vi "bumper e.vi"() -> ()   [LabVIEW 2013]
uses:
  <vilib>/NXT/Block Support/NXT_InputPort.ctl
  <vilib>/NXT/Block Support/NXT_MessageMailbox.ctl
  <vilib>/NXT/Subs/MotorOutput.ctl
  <vilib>/NXT/Block Support/NXT_OutputPort.ctl
  <vilib>/NXT/Dual Mode Library/Display/drawNumber.vi
  <vilib>/NXT/Dual Mode Library/BT/BlueTooth_Write_Num.vi
  <vilib>/NXT/Dual Mode Library/Display/drawNumber_float.vi
  <vilib>/NXT/NXTIO Xnodes/NXTIONodeSubVIs/NXTStopMotors.vi
  <vilib>/NXT/NXTIO Xnodes/AddressXNode/NXTIOAddress.xnode
  <vilib>/NXT/NXTIO Xnodes/NXTIOXNode/NXTIO.xnode
  <vilib>/NXT/Subs/LVHSConnector.ctl
  <vilib>/NXT/LegoClasses/BrickReference/BrickReference.lvclass
panel:
  out "Case Accord. BJr.":i32
  out "touch right":bool
  out "touch left":bool
  in  "threshold steer":dbl=0.2
  out "norm dist":dbl
  out "right dist":i16
  out "left dist":i16
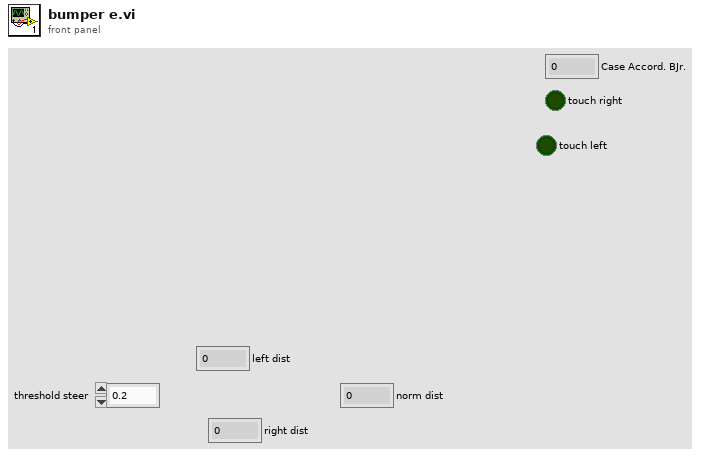
[diagram p1: front panel]
types:
  T1 = typedef "NXT_OutputPort.ctl" = u8
  T2 = typedef "NXT_MessageMailbox.ctl" = u8
  T3 = typedef "NXT_InputPort.ctl" = u32
  T4 = typedef "LVHSConnector.ctl" = refnum<class "BrickReference.lvclass">
  T5 = typedef "MotorOutput.ctl" = u8
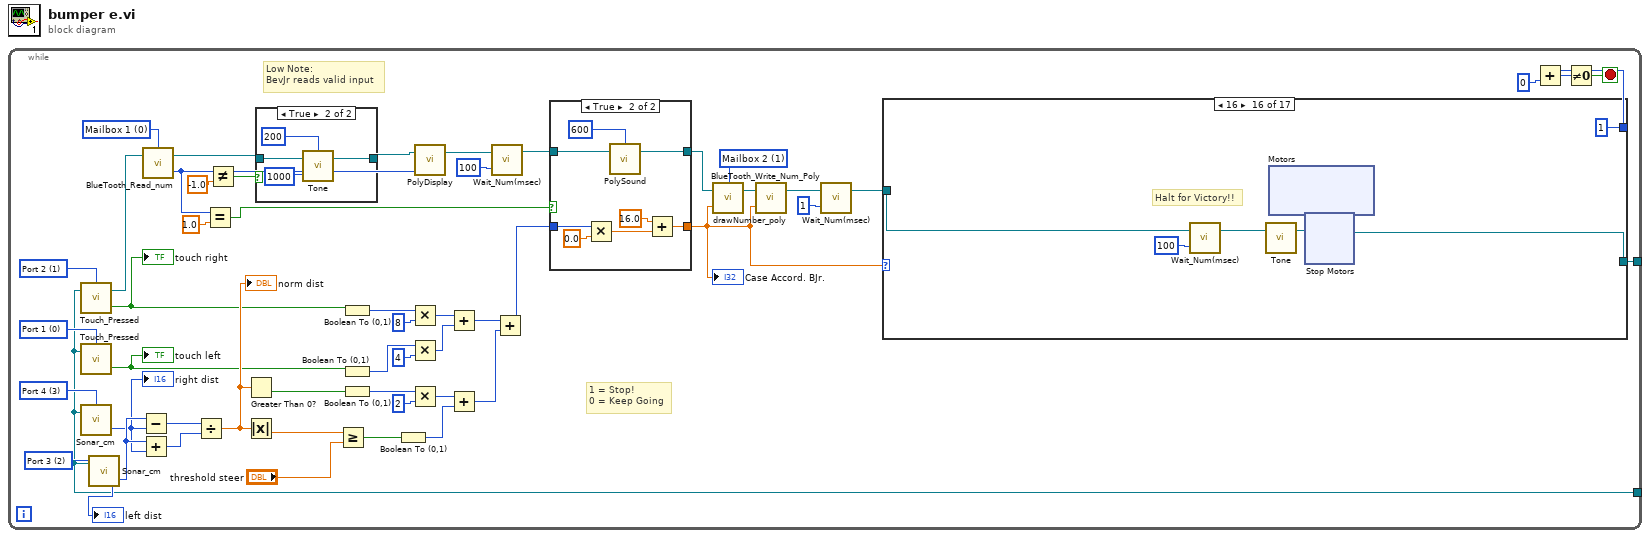
[diagram p0: block diagram]
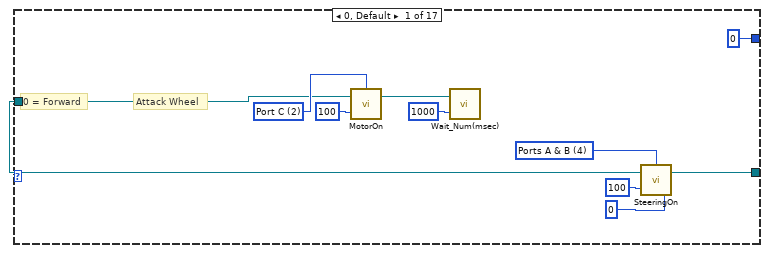
[diagram p3: hidden frame]
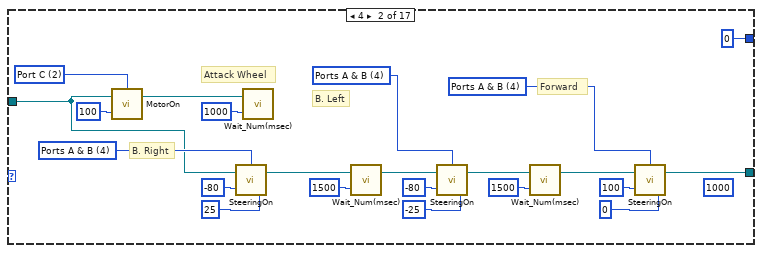
[diagram p4: hidden frame]
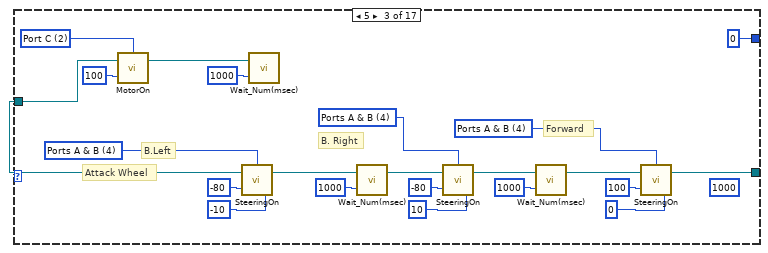
[diagram p5: hidden frame]
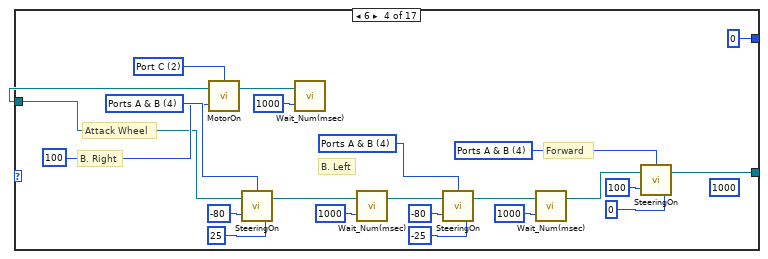
[diagram p6: hidden frame]
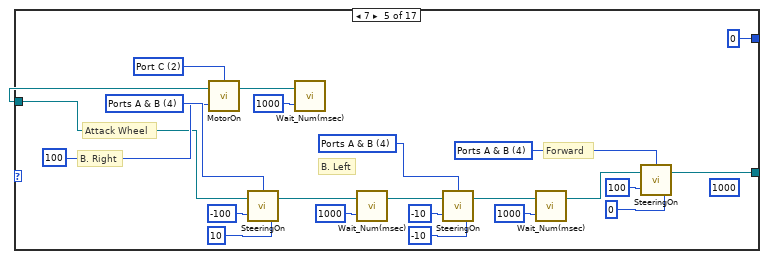
[diagram p7: hidden frame]
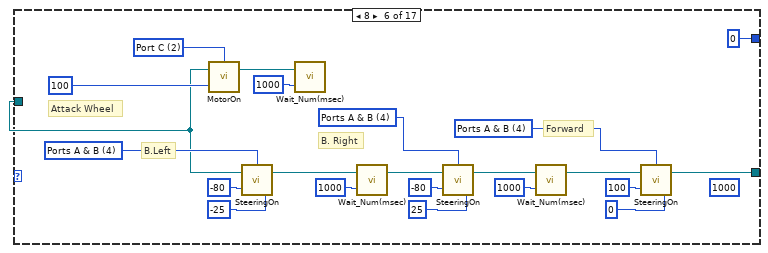
[diagram p8: hidden frame]
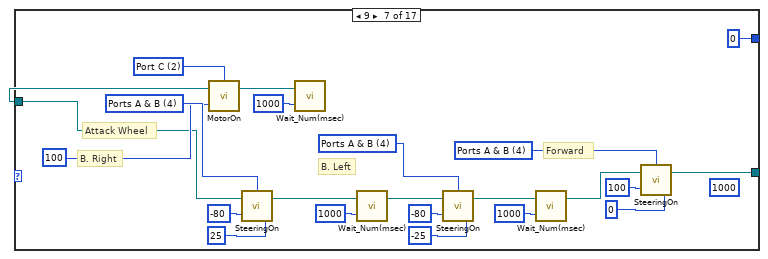
[diagram p9: hidden frame]
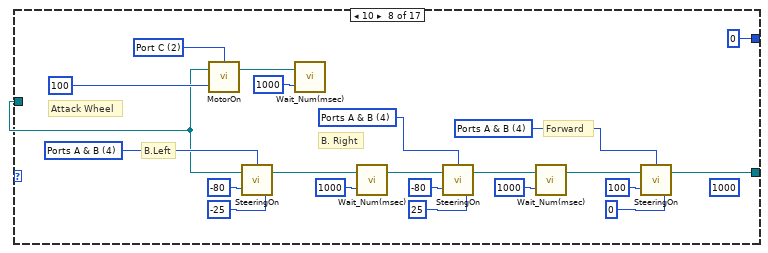
[diagram p10: hidden frame]
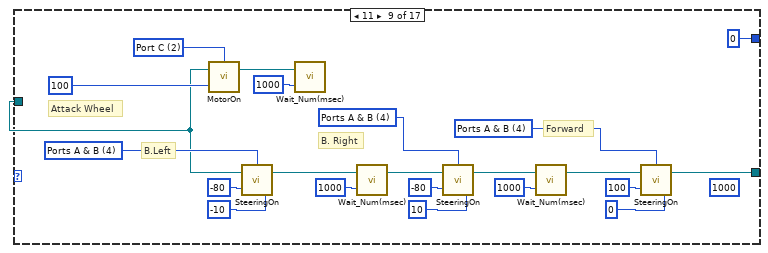
[diagram p11: hidden frame]
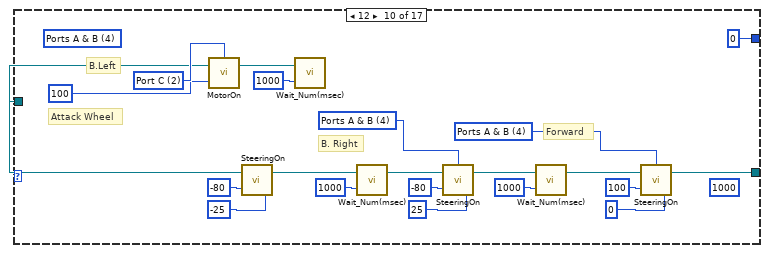
[diagram p12: hidden frame]
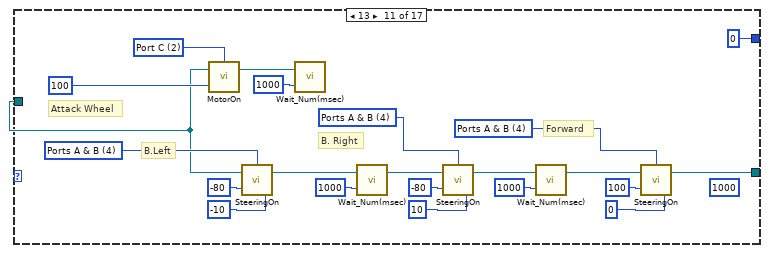
[diagram p13: hidden frame]
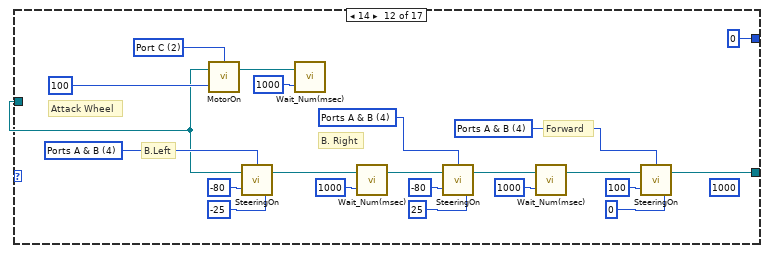
[diagram p14: hidden frame]
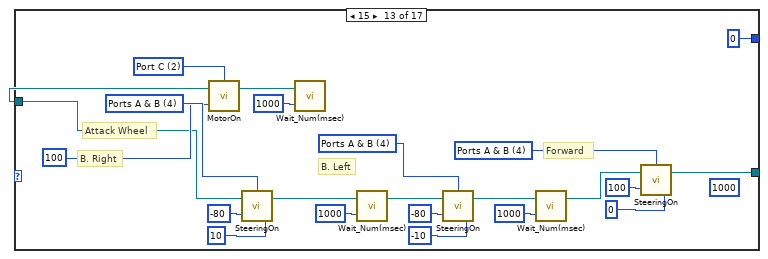
[diagram p15: hidden frame]
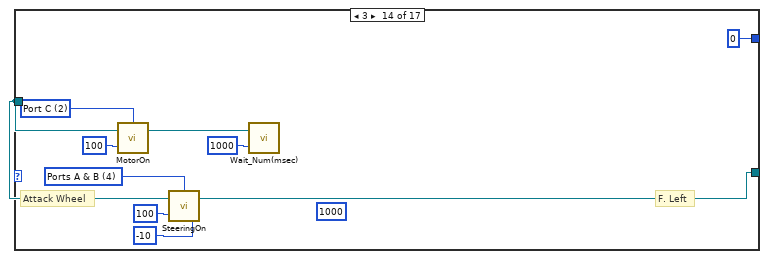
[diagram p16: hidden frame]
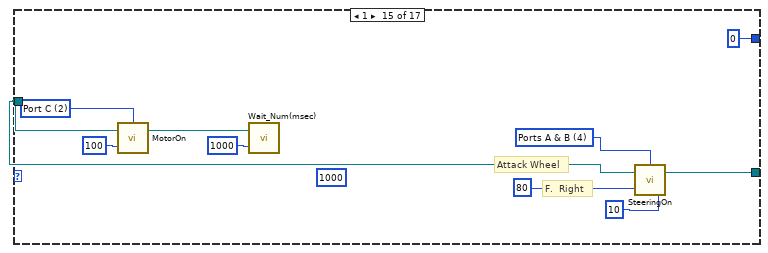
[diagram p17: hidden frame]
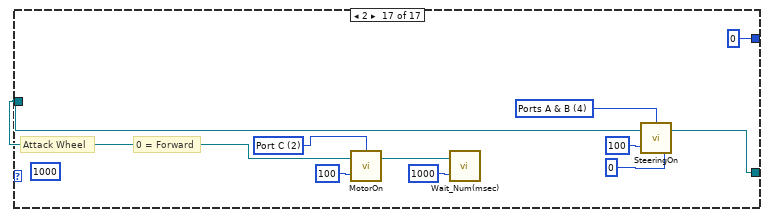
[diagram p18: hidden frame]
diagram:
  n1 = while {
    tunnel: [w20] -> _
    tunnel: [w14] -> _
    stop <- w22 stop-if-true
    w11 = T2 0 items=["Mailbox 1", "Mailbox 2", "Mailbox 3", "Mailbox 4", "Mailbox 5", "Mailbox 6", "Mailbox 7", "Mailbox 8", "Mailbox 9", "Mailbox 10"] ("Mailbox")
    w18 = T2 1 items=["Mailbox 1", "Mailbox 2", "Mailbox 3", "Mailbox 4", "Mailbox 5", "Mailbox 6", "Mailbox 7", "Mailbox 8", "Mailbox 9", "Mailbox 10"] ("Mailbox")
    w43 = T3 1 items=["Port 1", "Port 2", "Port 3", "Port 4"] ("Port (Port 1)")
    w44 = T3 0 items=["Port 1", "Port 2", "Port 3", "Port 4"] ("Port (Port 1)")
    w52 = T3 3 items=["Port 1", "Port 2", "Port 3", "Port 4"] ("Port (Port 4)")
    w53 = T3 2 items=["Port 1", "Port 2", "Port 3", "Port 4"] ("Port (Port 4)")
    # "Low Note:\nBevJr reads valid input"
    # "1 = Stop!\n0 = Keep Going"
    n2 = call <vilib>:"Sonar_cm.vi"("Port (Port 4)"=w53) -> ("Distance (cm)"=w51:i16, "NXT/EV3"=w20:T4)  [unwired: 2 in]
    "left dist" <- w51
    n3 = call <vilib>:"Touch_Pressed.vi"("NXT/EV3"=w20, "Port (Port 1)"=w43) -> ("Yes / No"=w29:bool, "NXT/EV3"=w10:T4)  [unwired: 1 in]
    "touch right" <- w29
    n4 = call <vilib>:"Touch_Pressed.vi"("NXT/EV3"=w20, "Port (Port 1)"=w44) -> ("Yes / No"=w30:bool)  [unwired: 1 in, 1 out]
    "touch left" <- w30
    n5 = call <vilib>:"Sonar_cm.vi"("NXT/EV3"=w20, "Port (Port 4)"=w52) -> ("Distance (cm)"=w50:i16)  [unwired: 1 in, 1 out]
    "right dist" <- w50
    n6 = Subtract(x=w51, y=w50) -> (x-y=w49:i16)
    n7 = Add(x=w51, y=w50) -> (x+y=w48:i16)
    n8 = call <vilib>:"BlueTooth_Read_num.vi"("NXT/EV3"=w10, "Mailbox"=w11) -> ("Message"=w4:i32, "NXT/EV3"=w3:T4)  [unwired: 1 in]
    n9 = Divide(x=w49, y=w48) -> (x/y=w45:dbl)
    "norm dist" <- w45
    n10 = Equal?(x=w4, y=1.0) -> (x = y?=w25:bool)
    n11 = Not Equal?(x=w4, y=-1.0) -> (x != y?=w5:bool)
    n12 = Greater Than 0?(x=w45) -> (x > 0?=w28:bool)
    n13 = Absolute Value(x=w45) -> (abs(x)=w47:dbl)
    n14 = case shown="True" w5 {
      tunnel: w3 -> [w54 w56]
      tunnel: [w54 w55] -> w2
      frame False {
      }
      frame True {
        n15 = call <vilib>:"Tone.vi"("Duration (500 ms)"=u16 1000, "NXT/EV3"=w56, "Tone (440 Hz)"=u16 200) -> ("NXT/EV3"=w55:T4)  [unwired: 1 in]
      }
    }
    n16 = Greater Or Equal?(x=w47, y="threshold steer") -> (x >= y?=w27:bool)
    n17 = Boolean To (0,1)(Boolean=w29) -> (0, 1=w38:i16)
    n18 = Boolean To (0,1)(Boolean=w30) -> (0, 1=w37:i16)
    n19 = Boolean To (0,1)(Boolean=w28) -> (0, 1=w42:i16)
    n20 = Boolean To (0,1)(Boolean=w27) -> (0, 1=w32:i16)
    n21 = Multiply(x=w38, y=i16 8) -> (x*y=w35:i16)
    n22 = Multiply(x=w37, y=i16 4) -> (x*y=w34:i16)
    n23 = Multiply(x=w42, y=i16 2) -> (x*y=w33:i16)
    n24 = call-poly <vilib>:"PolyDisplay.vi"("number"=w4, "NXT/EV3"=w2) -> ("NXT/EV3"=w12:T4)  [unwired: 2 in]
    n25 = Add(x=w35, y=w34) -> (x+y=w36:i16)
    n26 = Add(x=w33, y=w32) -> (x+y=w31:i16)
    n27 = call <vilib>:"Wait_Num(msec).vi"("Time (100 msec)"=u32 100, "NXT/EV3"=w12) -> ("NXT/EV3"=w9:T4)  [unwired: 2 in]
    n28 = Add(x=w36, y=w31) -> (x+y=w21:i16)
    n29 = case shown="True" w25 {
      tunnel: w21 -> [w376 w382]
      tunnel: [w376 w377] -> w7
      tunnel: w9 -> [w375 w381]
      tunnel: [w375 w380] -> w16
      frame False {
      }
      frame True {
        n30 = Multiply(x=w382, y=0.0) -> (x*y=w379:dbl)
        n31 = call-poly <vilib>:"PolySound.vi"("NXT/EV3"=w381, "Tone (440 Hz)"=u16 600) -> ("NXT/EV3"=w380:T4)  [unwired: 2 in]
        n32 = Add(x=16.0, y=w379) -> (x+y=w377:dbl)
      }
    }
    "Case Accord. BJr." <- w7
    n33 = call-poly <vilib>:"BlueTooth_Write_Num_Poly.vi"("Message"=w7, "NXT/EV3"=w16, "Mailbox"=w18) -> ("NXT/EV3"=w19:T4)  [unwired: 1 in]
    n34 = call-poly <vilib>:"drawNumber_poly.vi"("number"=w7, "NXT/EV3"=w19) -> ("NXT/EV3"=w1:T4)  [unwired: 2 in]
    n35 = call <vilib>:"Wait_Num(msec).vi"("Time (100 msec)"=u32 1, "NXT/EV3"=w1) -> ("NXT/EV3"=w15:T4)  [unwired: 2 in]
    n36 = case shown="16" w7 {
      tunnel: [w66 w84 w97 w119 w141 w172 w185 w207 w229 w251 w272 w294 w317 w339 w349 w356 w372] -> w14
      tunnel: w15 -> [w59 w69 w91 w113 w135 w157 w179 w201 w223 w245 w267 w288 w310 w332 w342 w352 w366]
      tunnel: [0 ("Steering (100)") 0 ("Steering (100)") 0 ("Steering (100)") 0 ("Steering (100)") 0 ("Steering (100)") 0 ("Steering (100)") 0 ("Steering (100)") 0 ("Steering (100)") 0 ("Steering (100)") 0 ("Steering (100)") 0 ("Steering (100)") 0 ("Steering (100)") 0 ("Steering (100)") 0 ("Steering (100)") 0 ("Steering (100)") 1 ("Steering (100)") 0 ("Steering (100)")] -> w13
      frame 0, Default {
        w64 = T5 2 items=["Port A"=0, "Port B"=1, "Port C"=2, "Ports A & B"=4, "Ports A & C"=5, "Ports B & C"=6, "All Ports"=3] ("Output Ports (A & B)")
        w65 = T5 4 items=["Port A"=0, "Port B"=1, "Port C"=2, "Ports A & B"=4, "Ports A & C"=5, "Ports B & C"=6, "All Ports"=3] ("Output Ports (A & B) 5")
        # "Attack Wheel"
        # "0 = Forward"
        n37 = call <vilib>:"MotorOn.vi"("Power (75)"=100, "NXT/EV3"=w59, "Output Port (All Ports)"=w64) -> ("NXT/EV3"=w62:T4)  [unwired: 1 in]
        n38 = call <vilib>:"Wait_Num(msec).vi"("Time (100 msec)"=u32 1000, "NXT/EV3"=w62) -> ()  [unwired: 2 in, 1 out]
        n39 = call <vilib>:"SteeringOn.vi"("Power (75)"=100, "Steering (100)"=0, "NXT/EV3"=w59, "Output Ports (A & B)"=w65) -> ("NXT/EV3"=w66:T4)
      }
      frame 4 {
        (unwired) u16 1000 ("Duration (500 ms)")
        w74 = T5 2 items=["Port A"=0, "Port B"=1, "Port C"=2, "Ports A & B"=4, "Ports A & C"=5, "Ports B & C"=6, "All Ports"=3] ("Output Ports (A & B)")
        w81 = T5 4 items=["Port A"=0, "Port B"=1, "Port C"=2, "Ports A & B"=4, "Ports A & C"=5, "Ports B & C"=6, "All Ports"=3] ("Output Ports (A & B) 15")
        w82 = T5 4 items=["Port A"=0, "Port B"=1, "Port C"=2, "Ports A & B"=4, "Ports A & C"=5, "Ports B & C"=6, "All Ports"=3] ("Output Port (All Ports) 6")
        w83 = T5 4 items=["Port A"=0, "Port B"=1, "Port C"=2, "Ports A & B"=4, "Ports A & C"=5, "Ports B & C"=6, "All Ports"=3] ("Output Ports (A & B) 16")
        # "Attack Wheel"
        # "Forward"
        # "B. Left"
        # "B. Right"
        n40 = call <vilib>:"MotorOn.vi"("Power (75)"=100, "NXT/EV3"=w69, "Output Port (All Ports)"=w74) -> ("NXT/EV3"=w72:T4)  [unwired: 1 in]
        n41 = call <vilib>:"SteeringOn.vi"("Power (75)"=-80, "Steering (100)"=25, "NXT/EV3"=w69, "Output Ports (A & B)"=w83) -> ("NXT/EV3"=w80:T4)
        n42 = call <vilib>:"Wait_Num(msec).vi"("Time (100 msec)"=u32 1000, "NXT/EV3"=w72) -> ()  [unwired: 2 in, 1 out]
        n43 = call <vilib>:"Wait_Num(msec).vi"("Time (100 msec)"=u32 1500, "NXT/EV3"=w80) -> ("NXT/EV3"=w79:T4)  [unwired: 2 in]
        n44 = call <vilib>:"SteeringOn.vi"("Power (75)"=-80, "Steering (100)"=-25, "NXT/EV3"=w79, "Output Ports (A & B)"=w82) -> ("NXT/EV3"=w78:T4)
        n45 = call <vilib>:"Wait_Num(msec).vi"("Time (100 msec)"=u32 1500, "NXT/EV3"=w78) -> ("NXT/EV3"=w77:T4)  [unwired: 2 in]
        n46 = call <vilib>:"SteeringOn.vi"("Power (75)"=100, "Steering (100)"=0, "NXT/EV3"=w77, "Output Ports (A & B)"=w81) -> ("NXT/EV3"=w84:T4)
      }
      frame 5 {
        (unwired) u16 1000 ("Duration (500 ms)")
        w96 = T5 2 items=["Port A"=0, "Port B"=1, "Port C"=2, "Ports A & B"=4, "Ports A & C"=5, "Ports B & C"=6, "All Ports"=3] ("Output Ports (A & B)")
        w104 = T5 4 items=["Port A"=0, "Port B"=1, "Port C"=2, "Ports A & B"=4, "Ports A & C"=5, "Ports B & C"=6, "All Ports"=3] ("Output Ports (A & B) 21")
        w105 = T5 4 items=["Port A"=0, "Port B"=1, "Port C"=2, "Ports A & B"=4, "Ports A & C"=5, "Ports B & C"=6, "All Ports"=3] ("Output Port (All Ports) 9")
        w106 = T5 4 items=["Port A"=0, "Port B"=1, "Port C"=2, "Ports A & B"=4, "Ports A & C"=5, "Ports B & C"=6, "All Ports"=3] ("Output Ports (A & B) 22")
        # "Attack Wheel"
        # "Forward"
        # "B. Right"
        # "B.Left"
        n47 = call <vilib>:"MotorOn.vi"("Power (75)"=100, "NXT/EV3"=w91, "Output Port (All Ports)"=w96) -> ("NXT/EV3"=w94:T4)  [unwired: 1 in]
        n48 = call <vilib>:"SteeringOn.vi"("Power (75)"=-80, "Steering (100)"=-10, "NXT/EV3"=w91, "Output Ports (A & B)"=w106) -> ("NXT/EV3"=w102:T4)
        n49 = call <vilib>:"Wait_Num(msec).vi"("Time (100 msec)"=u32 1000, "NXT/EV3"=w94) -> ()  [unwired: 2 in, 1 out]
        n50 = call <vilib>:"Wait_Num(msec).vi"("Time (100 msec)"=u32 1000, "NXT/EV3"=w102) -> ("NXT/EV3"=w101:T4)  [unwired: 2 in]
        n51 = call <vilib>:"SteeringOn.vi"("Power (75)"=-80, "Steering (100)"=10, "NXT/EV3"=w101, "Output Ports (A & B)"=w105) -> ("NXT/EV3"=w99:T4)
        n52 = call <vilib>:"Wait_Num(msec).vi"("Time (100 msec)"=u32 1000, "NXT/EV3"=w99) -> ("NXT/EV3"=w98:T4)  [unwired: 2 in]
        n53 = call <vilib>:"SteeringOn.vi"("Power (75)"=100, "Steering (100)"=0, "NXT/EV3"=w98, "Output Ports (A & B)"=w104) -> ("NXT/EV3"=w97:T4)
      }
      frame 6 {
        (unwired) u16 1000 ("Duration (500 ms)")
        w118 = T5 2 items=["Port A"=0, "Port B"=1, "Port C"=2, "Ports A & B"=4, "Ports A & C"=5, "Ports B & C"=6, "All Ports"=3] ("Output Ports (A & B)")
        w128 = T5 4 items=["Port A"=0, "Port B"=1, "Port C"=2, "Ports A & B"=4, "Ports A & C"=5, "Ports B & C"=6, "All Ports"=3] ("Output Ports (A & B) 15")
        w127 = T5 4 items=["Port A"=0, "Port B"=1, "Port C"=2, "Ports A & B"=4, "Ports A & C"=5, "Ports B & C"=6, "All Ports"=3] ("Output Port (All Ports) 6")
        w126 = T5 4 items=["Port A"=0, "Port B"=1, "Port C"=2, "Ports A & B"=4, "Ports A & C"=5, "Ports B & C"=6, "All Ports"=3] ("Output Ports (A & B) 16")
        # "Attack Wheel"
        # "Forward"
        # "B. Left"
        # "B. Right"
        n54 = call <vilib>:"MotorOn.vi"("Power (75)"=100, "NXT/EV3"=w113, "Output Port (All Ports)"=w118) -> ("NXT/EV3"=w116:T4)  [unwired: 1 in]
        n55 = call <vilib>:"SteeringOn.vi"("Power (75)"=-80, "Steering (100)"=25, "NXT/EV3"=w113, "Output Ports (A & B)"=w126) -> ("NXT/EV3"=w129:T4)
        n56 = call <vilib>:"Wait_Num(msec).vi"("Time (100 msec)"=u32 1000, "NXT/EV3"=w116) -> ()  [unwired: 2 in, 1 out]
        n57 = call <vilib>:"Wait_Num(msec).vi"("Time (100 msec)"=u32 1000, "NXT/EV3"=w129) -> ("NXT/EV3"=w130:T4)  [unwired: 2 in]
        n58 = call <vilib>:"SteeringOn.vi"("Power (75)"=-80, "Steering (100)"=-25, "NXT/EV3"=w130, "Output Ports (A & B)"=w127) -> ("NXT/EV3"=w131:T4)
        n59 = call <vilib>:"Wait_Num(msec).vi"("Time (100 msec)"=u32 1000, "NXT/EV3"=w131) -> ("NXT/EV3"=w132:T4)  [unwired: 2 in]
        n60 = call <vilib>:"SteeringOn.vi"("Power (75)"=100, "Steering (100)"=0, "NXT/EV3"=w132, "Output Ports (A & B)"=w128) -> ("NXT/EV3"=w119:T4)
      }
      frame 7 {
        (unwired) u16 1000 ("Duration (500 ms)")
        w140 = T5 2 items=["Port A"=0, "Port B"=1, "Port C"=2, "Ports A & B"=4, "Ports A & C"=5, "Ports B & C"=6, "All Ports"=3] ("Output Ports (A & B)")
        w150 = T5 4 items=["Port A"=0, "Port B"=1, "Port C"=2, "Ports A & B"=4, "Ports A & C"=5, "Ports B & C"=6, "All Ports"=3] ("Output Ports (A & B) 15")
        w149 = T5 4 items=["Port A"=0, "Port B"=1, "Port C"=2, "Ports A & B"=4, "Ports A & C"=5, "Ports B & C"=6, "All Ports"=3] ("Output Port (All Ports) 6")
        w148 = T5 4 items=["Port A"=0, "Port B"=1, "Port C"=2, "Ports A & B"=4, "Ports A & C"=5, "Ports B & C"=6, "All Ports"=3] ("Output Ports (A & B) 16")
        # "Attack Wheel"
        # "Forward"
        # "B. Left"
        # "B. Right"
        n61 = call <vilib>:"MotorOn.vi"("Power (75)"=100, "NXT/EV3"=w135, "Output Port (All Ports)"=w140) -> ("NXT/EV3"=w138:T4)  [unwired: 1 in]
        n62 = call <vilib>:"SteeringOn.vi"("Power (75)"=-100, "Steering (100)"=10, "NXT/EV3"=w135, "Output Ports (A & B)"=w148) -> ("NXT/EV3"=w151:T4)
        n63 = call <vilib>:"Wait_Num(msec).vi"("Time (100 msec)"=u32 1000, "NXT/EV3"=w138) -> ()  [unwired: 2 in, 1 out]
        n64 = call <vilib>:"Wait_Num(msec).vi"("Time (100 msec)"=u32 1000, "NXT/EV3"=w151) -> ("NXT/EV3"=w152:T4)  [unwired: 2 in]
        n65 = call <vilib>:"SteeringOn.vi"("Power (75)"=-10, "Steering (100)"=-10, "NXT/EV3"=w152, "Output Ports (A & B)"=w149) -> ("NXT/EV3"=w153:T4)
        n66 = call <vilib>:"Wait_Num(msec).vi"("Time (100 msec)"=u32 1000, "NXT/EV3"=w153) -> ("NXT/EV3"=w154:T4)  [unwired: 2 in]
        n67 = call <vilib>:"SteeringOn.vi"("Power (75)"=100, "Steering (100)"=0, "NXT/EV3"=w154, "Output Ports (A & B)"=w150) -> ("NXT/EV3"=w141:T4)
      }
      frame 8 {
        (unwired) u16 1000 ("Duration (500 ms)")
        w162 = T5 2 items=["Port A"=0, "Port B"=1, "Port C"=2, "Ports A & B"=4, "Ports A & C"=5, "Ports B & C"=6, "All Ports"=3] ("Output Ports (A & B)")
        w169 = T5 4 items=["Port A"=0, "Port B"=1, "Port C"=2, "Ports A & B"=4, "Ports A & C"=5, "Ports B & C"=6, "All Ports"=3] ("Output Ports (A & B) 21")
        w170 = T5 4 items=["Port A"=0, "Port B"=1, "Port C"=2, "Ports A & B"=4, "Ports A & C"=5, "Ports B & C"=6, "All Ports"=3] ("Output Port (All Ports) 9")
        w171 = T5 4 items=["Port A"=0, "Port B"=1, "Port C"=2, "Ports A & B"=4, "Ports A & C"=5, "Ports B & C"=6, "All Ports"=3] ("Output Ports (A & B) 22")
        # "Attack Wheel"
        # "Forward"
        # "B. Right"
        # "B.Left"
        n68 = call <vilib>:"MotorOn.vi"("Power (75)"=100, "NXT/EV3"=w157, "Output Port (All Ports)"=w162) -> ("NXT/EV3"=w160:T4)  [unwired: 1 in]
        n69 = call <vilib>:"SteeringOn.vi"("Power (75)"=-80, "Steering (100)"=-25, "NXT/EV3"=w157, "Output Ports (A & B)"=w171) -> ("NXT/EV3"=w167:T4)
        n70 = call <vilib>:"Wait_Num(msec).vi"("Time (100 msec)"=u32 1000, "NXT/EV3"=w160) -> ()  [unwired: 2 in, 1 out]
        n71 = call <vilib>:"Wait_Num(msec).vi"("Time (100 msec)"=u32 1000, "NXT/EV3"=w167) -> ("NXT/EV3"=w166:T4)  [unwired: 2 in]
        n72 = call <vilib>:"SteeringOn.vi"("Power (75)"=-80, "Steering (100)"=25, "NXT/EV3"=w166, "Output Ports (A & B)"=w170) -> ("NXT/EV3"=w164:T4)
        n73 = call <vilib>:"Wait_Num(msec).vi"("Time (100 msec)"=u32 1000, "NXT/EV3"=w164) -> ("NXT/EV3"=w163:T4)  [unwired: 2 in]
        n74 = call <vilib>:"SteeringOn.vi"("Power (75)"=100, "Steering (100)"=0, "NXT/EV3"=w163, "Output Ports (A & B)"=w169) -> ("NXT/EV3"=w172:T4)
      }
      frame 9 {
        (unwired) u16 1000 ("Duration (500 ms)")
        w184 = T5 2 items=["Port A"=0, "Port B"=1, "Port C"=2, "Ports A & B"=4, "Ports A & C"=5, "Ports B & C"=6, "All Ports"=3] ("Output Ports (A & B)")
        w192 = T5 4 items=["Port A"=0, "Port B"=1, "Port C"=2, "Ports A & B"=4, "Ports A & C"=5, "Ports B & C"=6, "All Ports"=3] ("Output Ports (A & B) 15")
        w193 = T5 4 items=["Port A"=0, "Port B"=1, "Port C"=2, "Ports A & B"=4, "Ports A & C"=5, "Ports B & C"=6, "All Ports"=3] ("Output Port (All Ports) 6")
        w194 = T5 4 items=["Port A"=0, "Port B"=1, "Port C"=2, "Ports A & B"=4, "Ports A & C"=5, "Ports B & C"=6, "All Ports"=3] ("Output Ports (A & B) 16")
        # "Attack Wheel"
        # "Forward"
        # "B. Left"
        # "B. Right"
        n75 = call <vilib>:"MotorOn.vi"("Power (75)"=100, "NXT/EV3"=w179, "Output Port (All Ports)"=w184) -> ("NXT/EV3"=w182:T4)  [unwired: 1 in]
        n76 = call <vilib>:"SteeringOn.vi"("Power (75)"=-80, "Steering (100)"=25, "NXT/EV3"=w179, "Output Ports (A & B)"=w194) -> ("NXT/EV3"=w191:T4)
        n77 = call <vilib>:"Wait_Num(msec).vi"("Time (100 msec)"=u32 1000, "NXT/EV3"=w182) -> ()  [unwired: 2 in, 1 out]
        n78 = call <vilib>:"Wait_Num(msec).vi"("Time (100 msec)"=u32 1000, "NXT/EV3"=w191) -> ("NXT/EV3"=w190:T4)  [unwired: 2 in]
        n79 = call <vilib>:"SteeringOn.vi"("Power (75)"=-80, "Steering (100)"=-25, "NXT/EV3"=w190, "Output Ports (A & B)"=w193) -> ("NXT/EV3"=w189:T4)
        n80 = call <vilib>:"Wait_Num(msec).vi"("Time (100 msec)"=u32 1000, "NXT/EV3"=w189) -> ("NXT/EV3"=w188:T4)  [unwired: 2 in]
        n81 = call <vilib>:"SteeringOn.vi"("Power (75)"=100, "Steering (100)"=0, "NXT/EV3"=w188, "Output Ports (A & B)"=w192) -> ("NXT/EV3"=w185:T4)
      }
      frame 10 {
        (unwired) u16 1000 ("Duration (500 ms)")
        w206 = T5 2 items=["Port A"=0, "Port B"=1, "Port C"=2, "Ports A & B"=4, "Ports A & C"=5, "Ports B & C"=6, "All Ports"=3] ("Output Ports (A & B)")
        w216 = T5 4 items=["Port A"=0, "Port B"=1, "Port C"=2, "Ports A & B"=4, "Ports A & C"=5, "Ports B & C"=6, "All Ports"=3] ("Output Ports (A & B) 21")
        w215 = T5 4 items=["Port A"=0, "Port B"=1, "Port C"=2, "Ports A & B"=4, "Ports A & C"=5, "Ports B & C"=6, "All Ports"=3] ("Output Port (All Ports) 9")
        w214 = T5 4 items=["Port A"=0, "Port B"=1, "Port C"=2, "Ports A & B"=4, "Ports A & C"=5, "Ports B & C"=6, "All Ports"=3] ("Output Ports (A & B) 22")
        # "Attack Wheel"
        # "Forward"
        # "B. Right"
        # "B.Left"
        n82 = call <vilib>:"MotorOn.vi"("Power (75)"=100, "NXT/EV3"=w201, "Output Port (All Ports)"=w206) -> ("NXT/EV3"=w204:T4)  [unwired: 1 in]
        n83 = call <vilib>:"SteeringOn.vi"("Power (75)"=-80, "Steering (100)"=-25, "NXT/EV3"=w201, "Output Ports (A & B)"=w214) -> ("NXT/EV3"=w218:T4)
        n84 = call <vilib>:"Wait_Num(msec).vi"("Time (100 msec)"=u32 1000, "NXT/EV3"=w204) -> ()  [unwired: 2 in, 1 out]
        n85 = call <vilib>:"Wait_Num(msec).vi"("Time (100 msec)"=u32 1000, "NXT/EV3"=w218) -> ("NXT/EV3"=w219:T4)  [unwired: 2 in]
        n86 = call <vilib>:"SteeringOn.vi"("Power (75)"=-80, "Steering (100)"=25, "NXT/EV3"=w219, "Output Ports (A & B)"=w215) -> ("NXT/EV3"=w221:T4)
        n87 = call <vilib>:"Wait_Num(msec).vi"("Time (100 msec)"=u32 1000, "NXT/EV3"=w221) -> ("NXT/EV3"=w222:T4)  [unwired: 2 in]
        n88 = call <vilib>:"SteeringOn.vi"("Power (75)"=100, "Steering (100)"=0, "NXT/EV3"=w222, "Output Ports (A & B)"=w216) -> ("NXT/EV3"=w207:T4)
      }
      frame 11 {
        (unwired) u16 1000 ("Duration (500 ms)")
        w228 = T5 2 items=["Port A"=0, "Port B"=1, "Port C"=2, "Ports A & B"=4, "Ports A & C"=5, "Ports B & C"=6, "All Ports"=3] ("Output Ports (A & B)")
        w238 = T5 4 items=["Port A"=0, "Port B"=1, "Port C"=2, "Ports A & B"=4, "Ports A & C"=5, "Ports B & C"=6, "All Ports"=3] ("Output Ports (A & B) 21")
        w237 = T5 4 items=["Port A"=0, "Port B"=1, "Port C"=2, "Ports A & B"=4, "Ports A & C"=5, "Ports B & C"=6, "All Ports"=3] ("Output Port (All Ports) 9")
        w236 = T5 4 items=["Port A"=0, "Port B"=1, "Port C"=2, "Ports A & B"=4, "Ports A & C"=5, "Ports B & C"=6, "All Ports"=3] ("Output Ports (A & B) 22")
        # "Attack Wheel"
        # "Forward"
        # "B. Right"
        # "B.Left"
        n89 = call <vilib>:"MotorOn.vi"("Power (75)"=100, "NXT/EV3"=w223, "Output Port (All Ports)"=w228) -> ("NXT/EV3"=w226:T4)  [unwired: 1 in]
        n90 = call <vilib>:"SteeringOn.vi"("Power (75)"=-80, "Steering (100)"=-10, "NXT/EV3"=w223, "Output Ports (A & B)"=w236) -> ("NXT/EV3"=w240:T4)
        n91 = call <vilib>:"Wait_Num(msec).vi"("Time (100 msec)"=u32 1000, "NXT/EV3"=w226) -> ()  [unwired: 2 in, 1 out]
        n92 = call <vilib>:"Wait_Num(msec).vi"("Time (100 msec)"=u32 1000, "NXT/EV3"=w240) -> ("NXT/EV3"=w241:T4)  [unwired: 2 in]
        n93 = call <vilib>:"SteeringOn.vi"("Power (75)"=-80, "Steering (100)"=10, "NXT/EV3"=w241, "Output Ports (A & B)"=w237) -> ("NXT/EV3"=w243:T4)
        n94 = call <vilib>:"Wait_Num(msec).vi"("Time (100 msec)"=u32 1000, "NXT/EV3"=w243) -> ("NXT/EV3"=w244:T4)  [unwired: 2 in]
        n95 = call <vilib>:"SteeringOn.vi"("Power (75)"=100, "Steering (100)"=0, "NXT/EV3"=w244, "Output Ports (A & B)"=w238) -> ("NXT/EV3"=w229:T4)
      }
      frame 12 {
        (unwired) u16 1000 ("Duration (500 ms)")
        w250 = T5 2 items=["Port A"=0, "Port B"=1, "Port C"=2, "Ports A & B"=4, "Ports A & C"=5, "Ports B & C"=6, "All Ports"=3] ("Output Ports (A & B)")
        w259 = T5 4 items=["Port A"=0, "Port B"=1, "Port C"=2, "Ports A & B"=4, "Ports A & C"=5, "Ports B & C"=6, "All Ports"=3] ("Output Ports (A & B) 21")
        w258 = T5 4 items=["Port A"=0, "Port B"=1, "Port C"=2, "Ports A & B"=4, "Ports A & C"=5, "Ports B & C"=6, "All Ports"=3] ("Output Port (All Ports) 9")
        (unwired) T5 4 items=["Port A"=0, "Port B"=1, "Port C"=2, "Ports A & B"=4, "Ports A & C"=5, "Ports B & C"=6, "All Ports"=3] ("Output Ports (A & B) 22")
        # "Attack Wheel"
        # "Forward"
        # "B. Right"
        # "B.Left"
        n96 = call <vilib>:"MotorOn.vi"("Power (75)"=100, "NXT/EV3"=w245, "Output Port (All Ports)"=w250) -> ("NXT/EV3"=w248:T4)  [unwired: 1 in]
        n97 = call <vilib>:"SteeringOn.vi"("Power (75)"=-80, "Steering (100)"=-25, "NXT/EV3"=w245) -> ("NXT/EV3"=w261:T4)  [unwired: 1 in]
        n98 = call <vilib>:"Wait_Num(msec).vi"("Time (100 msec)"=u32 1000, "NXT/EV3"=w248) -> ()  [unwired: 2 in, 1 out]
        n99 = call <vilib>:"Wait_Num(msec).vi"("Time (100 msec)"=u32 1000, "NXT/EV3"=w261) -> ("NXT/EV3"=w262:T4)  [unwired: 2 in]
        n100 = call <vilib>:"SteeringOn.vi"("Power (75)"=-80, "Steering (100)"=25, "NXT/EV3"=w262, "Output Ports (A & B)"=w258) -> ("NXT/EV3"=w264:T4)
        n101 = call <vilib>:"Wait_Num(msec).vi"("Time (100 msec)"=u32 1000, "NXT/EV3"=w264) -> ("NXT/EV3"=w265:T4)  [unwired: 2 in]
        n102 = call <vilib>:"SteeringOn.vi"("Power (75)"=100, "Steering (100)"=0, "NXT/EV3"=w265, "Output Ports (A & B)"=w259) -> ("NXT/EV3"=w251:T4)
      }
      frame 13 {
        (unwired) u16 1000 ("Duration (500 ms)")
        w271 = T5 2 items=["Port A"=0, "Port B"=1, "Port C"=2, "Ports A & B"=4, "Ports A & C"=5, "Ports B & C"=6, "All Ports"=3] ("Output Ports (A & B)")
        w279 = T5 4 items=["Port A"=0, "Port B"=1, "Port C"=2, "Ports A & B"=4, "Ports A & C"=5, "Ports B & C"=6, "All Ports"=3] ("Output Ports (A & B) 21")
        w280 = T5 4 items=["Port A"=0, "Port B"=1, "Port C"=2, "Ports A & B"=4, "Ports A & C"=5, "Ports B & C"=6, "All Ports"=3] ("Output Port (All Ports) 9")
        w281 = T5 4 items=["Port A"=0, "Port B"=1, "Port C"=2, "Ports A & B"=4, "Ports A & C"=5, "Ports B & C"=6, "All Ports"=3] ("Output Ports (A & B) 22")
        # "Attack Wheel"
        # "Forward"
        # "B. Right"
        # "B.Left"
        n103 = call <vilib>:"MotorOn.vi"("Power (75)"=100, "NXT/EV3"=w267, "Output Port (All Ports)"=w271) -> ("NXT/EV3"=w269:T4)  [unwired: 1 in]
        n104 = call <vilib>:"SteeringOn.vi"("Power (75)"=-80, "Steering (100)"=-10, "NXT/EV3"=w267, "Output Ports (A & B)"=w281) -> ("NXT/EV3"=w277:T4)
        n105 = call <vilib>:"Wait_Num(msec).vi"("Time (100 msec)"=u32 1000, "NXT/EV3"=w269) -> ()  [unwired: 2 in, 1 out]
        n106 = call <vilib>:"Wait_Num(msec).vi"("Time (100 msec)"=u32 1000, "NXT/EV3"=w277) -> ("NXT/EV3"=w276:T4)  [unwired: 2 in]
        n107 = call <vilib>:"SteeringOn.vi"("Power (75)"=-80, "Steering (100)"=10, "NXT/EV3"=w276, "Output Ports (A & B)"=w280) -> ("NXT/EV3"=w274:T4)
        n108 = call <vilib>:"Wait_Num(msec).vi"("Time (100 msec)"=u32 1000, "NXT/EV3"=w274) -> ("NXT/EV3"=w273:T4)  [unwired: 2 in]
        n109 = call <vilib>:"SteeringOn.vi"("Power (75)"=100, "Steering (100)"=0, "NXT/EV3"=w273, "Output Ports (A & B)"=w279) -> ("NXT/EV3"=w272:T4)
      }
      frame 14 {
        (unwired) u16 1000 ("Duration (500 ms)")
        w293 = T5 2 items=["Port A"=0, "Port B"=1, "Port C"=2, "Ports A & B"=4, "Ports A & C"=5, "Ports B & C"=6, "All Ports"=3] ("Output Ports (A & B)")
        w303 = T5 4 items=["Port A"=0, "Port B"=1, "Port C"=2, "Ports A & B"=4, "Ports A & C"=5, "Ports B & C"=6, "All Ports"=3] ("Output Ports (A & B) 21")
        w302 = T5 4 items=["Port A"=0, "Port B"=1, "Port C"=2, "Ports A & B"=4, "Ports A & C"=5, "Ports B & C"=6, "All Ports"=3] ("Output Port (All Ports) 9")
        w301 = T5 4 items=["Port A"=0, "Port B"=1, "Port C"=2, "Ports A & B"=4, "Ports A & C"=5, "Ports B & C"=6, "All Ports"=3] ("Output Ports (A & B) 22")
        # "Attack Wheel"
        # "Forward"
        # "B. Right"
        # "B.Left"
        n110 = call <vilib>:"MotorOn.vi"("Power (75)"=100, "NXT/EV3"=w288, "Output Port (All Ports)"=w293) -> ("NXT/EV3"=w291:T4)  [unwired: 1 in]
        n111 = call <vilib>:"SteeringOn.vi"("Power (75)"=-80, "Steering (100)"=-25, "NXT/EV3"=w288, "Output Ports (A & B)"=w301) -> ("NXT/EV3"=w305:T4)
        n112 = call <vilib>:"Wait_Num(msec).vi"("Time (100 msec)"=u32 1000, "NXT/EV3"=w291) -> ()  [unwired: 2 in, 1 out]
        n113 = call <vilib>:"Wait_Num(msec).vi"("Time (100 msec)"=u32 1000, "NXT/EV3"=w305) -> ("NXT/EV3"=w306:T4)  [unwired: 2 in]
        n114 = call <vilib>:"SteeringOn.vi"("Power (75)"=-80, "Steering (100)"=25, "NXT/EV3"=w306, "Output Ports (A & B)"=w302) -> ("NXT/EV3"=w308:T4)
        n115 = call <vilib>:"Wait_Num(msec).vi"("Time (100 msec)"=u32 1000, "NXT/EV3"=w308) -> ("NXT/EV3"=w309:T4)  [unwired: 2 in]
        n116 = call <vilib>:"SteeringOn.vi"("Power (75)"=100, "Steering (100)"=0, "NXT/EV3"=w309, "Output Ports (A & B)"=w303) -> ("NXT/EV3"=w294:T4)
      }
      frame 15 {
        (unwired) u16 1000 ("Duration (500 ms)")
        w315 = T5 2 items=["Port A"=0, "Port B"=1, "Port C"=2, "Ports A & B"=4, "Ports A & C"=5, "Ports B & C"=6, "All Ports"=3] ("Output Ports (A & B)")
        w324 = T5 4 items=["Port A"=0, "Port B"=1, "Port C"=2, "Ports A & B"=4, "Ports A & C"=5, "Ports B & C"=6, "All Ports"=3] ("Output Ports (A & B) 15")
        w325 = T5 4 items=["Port A"=0, "Port B"=1, "Port C"=2, "Ports A & B"=4, "Ports A & C"=5, "Ports B & C"=6, "All Ports"=3] ("Output Port (All Ports) 6")
        w316 = T5 4 items=["Port A"=0, "Port B"=1, "Port C"=2, "Ports A & B"=4, "Ports A & C"=5, "Ports B & C"=6, "All Ports"=3] ("Output Ports (A & B) 16")
        # "Attack Wheel"
        # "Forward"
        # "B. Left"
        # "B. Right"
        n117 = call <vilib>:"MotorOn.vi"("Power (75)"=100, "NXT/EV3"=w310, "Output Port (All Ports)"=w315) -> ("NXT/EV3"=w313:T4)  [unwired: 1 in]
        n118 = call <vilib>:"SteeringOn.vi"("Power (75)"=-80, "Steering (100)"=10, "NXT/EV3"=w310, "Output Ports (A & B)"=w316) -> ("NXT/EV3"=w323:T4)
        n119 = call <vilib>:"Wait_Num(msec).vi"("Time (100 msec)"=u32 1000, "NXT/EV3"=w313) -> ()  [unwired: 2 in, 1 out]
        n120 = call <vilib>:"Wait_Num(msec).vi"("Time (100 msec)"=u32 1000, "NXT/EV3"=w323) -> ("NXT/EV3"=w322:T4)  [unwired: 2 in]
        n121 = call <vilib>:"SteeringOn.vi"("Power (75)"=-80, "Steering (100)"=-10, "NXT/EV3"=w322, "Output Ports (A & B)"=w325) -> ("NXT/EV3"=w321:T4)
        n122 = call <vilib>:"Wait_Num(msec).vi"("Time (100 msec)"=u32 1000, "NXT/EV3"=w321) -> ("NXT/EV3"=w320:T4)  [unwired: 2 in]
        n123 = call <vilib>:"SteeringOn.vi"("Power (75)"=100, "Steering (100)"=0, "NXT/EV3"=w320, "Output Ports (A & B)"=w324) -> ("NXT/EV3"=w317:T4)
      }
      frame 3 {
        (unwired) u16 1000 ("Duration (500 ms)")
        w337 = T5 2 items=["Port A"=0, "Port B"=1, "Port C"=2, "Ports A & B"=4, "Ports A & C"=5, "Ports B & C"=6, "All Ports"=3] ("Output Ports (A & B)")
        w338 = T5 4 items=["Port A"=0, "Port B"=1, "Port C"=2, "Ports A & B"=4, "Ports A & C"=5, "Ports B & C"=6, "All Ports"=3] ("Output Port (All Ports) 3")
        # "Attack Wheel"
        # "F. Left"
        n124 = call <vilib>:"MotorOn.vi"("Power (75)"=100, "NXT/EV3"=w332, "Output Port (All Ports)"=w337) -> ("NXT/EV3"=w335:T4)  [unwired: 1 in]
        n125 = call <vilib>:"SteeringOn.vi"("Power (75)"=100, "Steering (100)"=-10, "NXT/EV3"=w332, "Output Ports (A & B)"=w338) -> ("NXT/EV3"=w339:T4)
        n126 = call <vilib>:"Wait_Num(msec).vi"("Time (100 msec)"=u32 1000, "NXT/EV3"=w335) -> ()  [unwired: 2 in, 1 out]
      }
      frame 1 {
        (unwired) u16 1000 ("Duration (500 ms)")
        w347 = T5 2 items=["Port A"=0, "Port B"=1, "Port C"=2, "Ports A & B"=4, "Ports A & C"=5, "Ports B & C"=6, "All Ports"=3] ("Output Ports (A & B)")
        w348 = T5 4 items=["Port A"=0, "Port B"=1, "Port C"=2, "Ports A & B"=4, "Ports A & C"=5, "Ports B & C"=6, "All Ports"=3] ("Output Ports (A & B) 12")
        # "Attack Wheel"
        # "F.  Right"
        n127 = call <vilib>:"MotorOn.vi"("Power (75)"=100, "NXT/EV3"=w342, "Output Port (All Ports)"=w347) -> ("NXT/EV3"=w345:T4)  [unwired: 1 in]
        n128 = call <vilib>:"Wait_Num(msec).vi"("Time (100 msec)"=u32 1000, "NXT/EV3"=w345) -> ()  [unwired: 2 in, 1 out]
        n129 = call <vilib>:"SteeringOn.vi"("Power (75)"=80, "Steering (100)"=10, "NXT/EV3"=w342, "Output Ports (A & B)"=w348) -> ("NXT/EV3"=w349:T4)
      }
      frame 16 {
        # "Halt for Victory!!"
        n130 = call <vilib>:"Wait_Num(msec).vi"("Time (100 msec)"=u32 100, "NXT/EV3"=w352) -> ("NXT/EV3"=w355:T4)  [unwired: 2 in]
        n131 = call <vilib>:"Tone.vi"("NXT/EV3"=w355) -> ("NXT/EV3"=w354:T4)  [unwired: 3 in]
        n132 = xnode "Motors"() -> ("Motor"=w358:cluster{"Port":T1, "Port":T1})
        n133 = xnode "Stop Motors"("Motors"=w358, "NXT/EV3"=w354) -> ("NXT/EV3"=w356:T4)
      }
      frame 2 {
        (unwired) u16 1000 ("Duration (500 ms)")
        w370 = T5 2 items=["Port A"=0, "Port B"=1, "Port C"=2, "Ports A & B"=4, "Ports A & C"=5, "Ports B & C"=6, "All Ports"=3] ("Output Ports (A & B)")
        w371 = T5 4 items=["Port A"=0, "Port B"=1, "Port C"=2, "Ports A & B"=4, "Ports A & C"=5, "Ports B & C"=6, "All Ports"=3] ("Output Ports (A & B) 10")
        # "Attack Wheel"
        # "0 = Forward"
        n134 = call <vilib>:"MotorOn.vi"("Power (75)"=100, "NXT/EV3"=w366, "Output Port (All Ports)"=w370) -> ("NXT/EV3"=w368:T4)  [unwired: 1 in]
        n135 = call <vilib>:"Wait_Num(msec).vi"("Time (100 msec)"=u32 1000, "NXT/EV3"=w368) -> ()  [unwired: 2 in, 1 out]
        n136 = call <vilib>:"SteeringOn.vi"("Power (75)"=100, "Steering (100)"=0, "NXT/EV3"=w366, "Output Ports (A & B)"=w371) -> ("NXT/EV3"=w372:T4)
      }
    }
    n137 = Add(x=w13, y=0) -> (x+y=w23:i32)
    n138 = Not Equal To 0?(x=w23) -> (x != 0?=w22:bool)
  }
